vi "PrgEditor.vi"() -> ()   [LabVIEW 2012, in "StimulCtrls.lvlib"]
uses:
  StimulCtrls.lvlib
  SEQPanel.ctl
  Time Slider/Time Slider.xctl
panel:
  in  "Stop Button":bool
  in  "Range Max":dbl=100.0 min=0.0 step=10.0
  in  "Range Min":dbl
  in  "Programs":T1
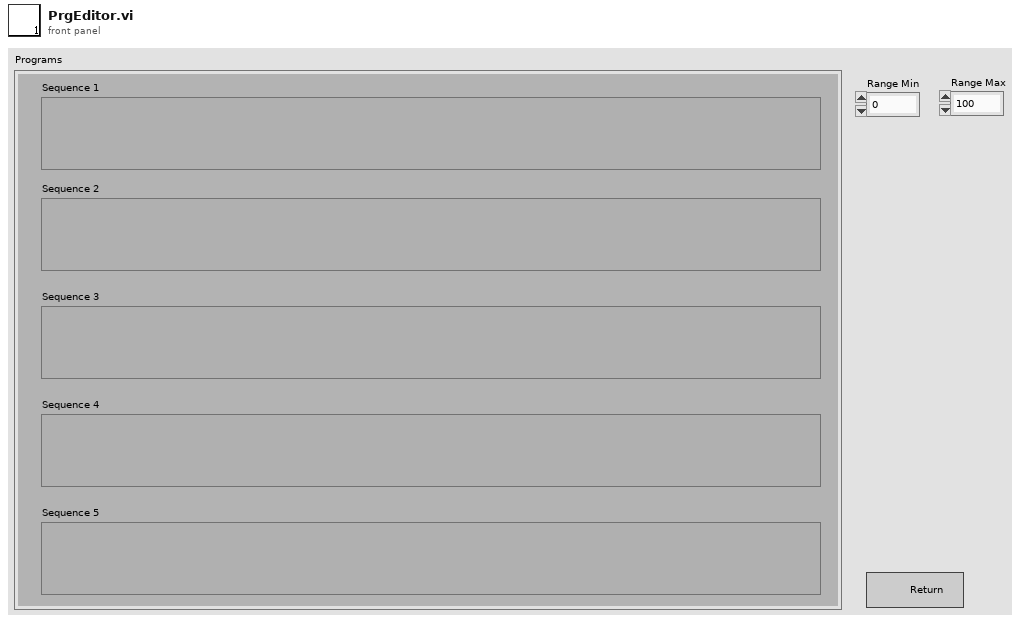
[diagram p1: front panel]
types:
  T1 = typedef "StimulCtrls.lvlib/SEQPanel.ctl" = cluster{"Sequence 1":cluster{"Data":dbl, "Data 2":dbl, "Data 3":dbl}, "Sequence 2":cluster{"Data":dbl, "Data 2":dbl, "Data 3":dbl}, "Sequence 3":cluster{"Data":dbl, "Data 2":dbl, "Data 3":dbl}, "Sequence 4":cluster{"Data":dbl, "Data 2":dbl, "Data 3":dbl}, "Sequence 5":cluster{"Data":dbl, "Data 2":dbl, "Data 3":dbl}}
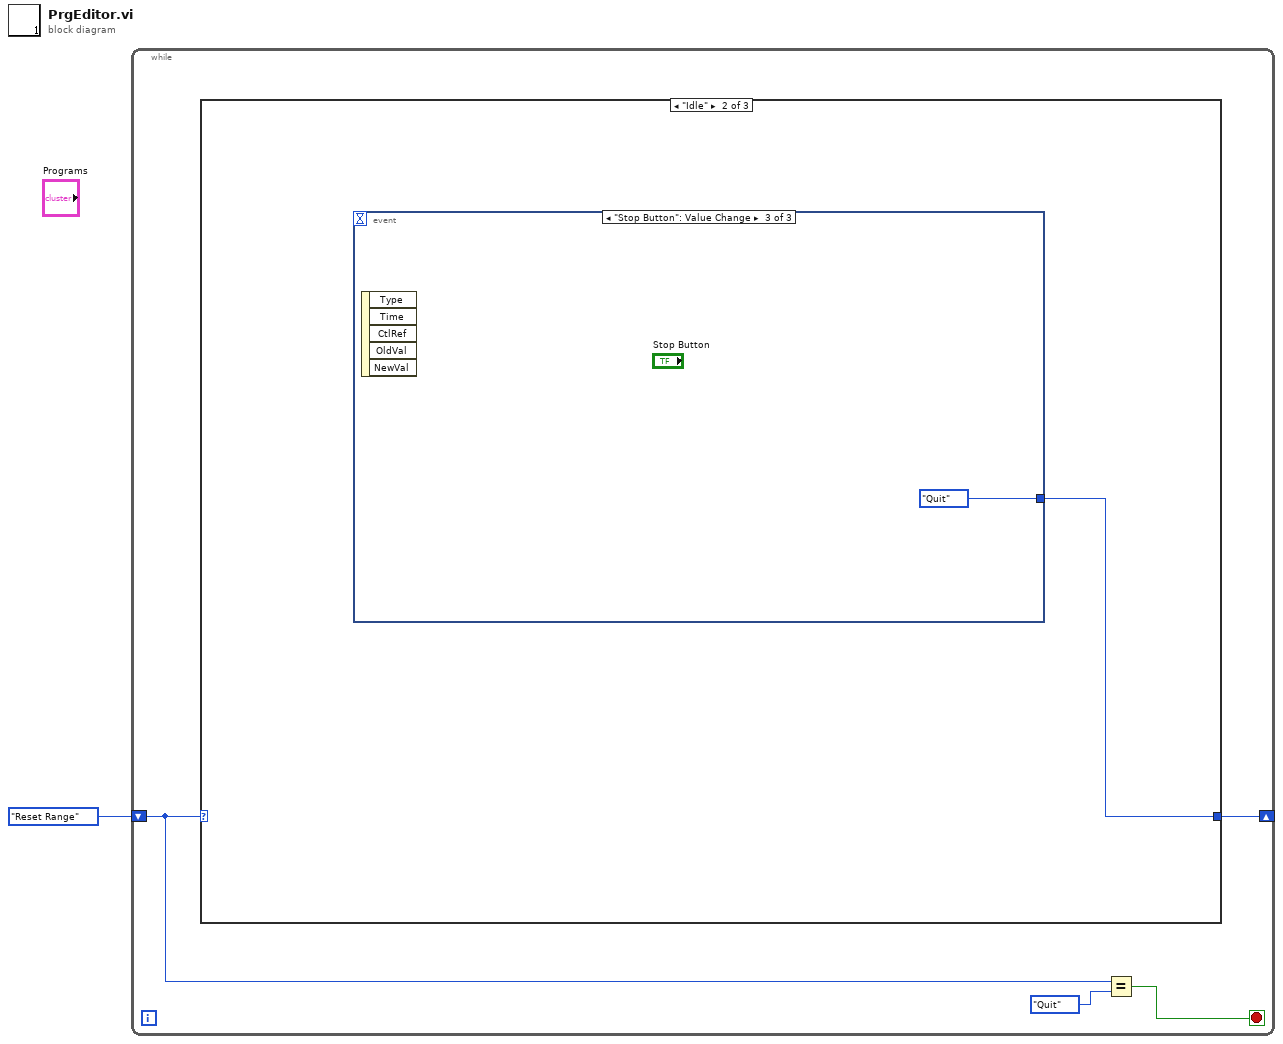
[diagram p0: block diagram]
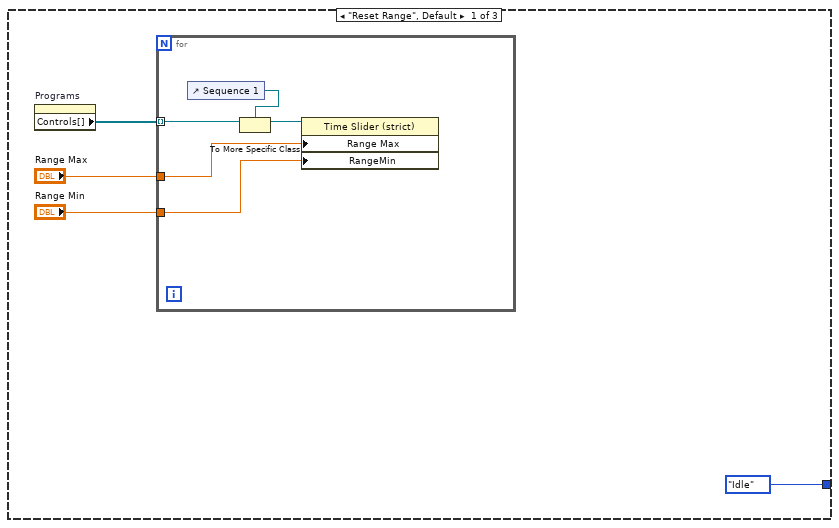
[diagram p2: hidden frame]
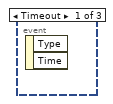
[diagram p3: hidden frame]
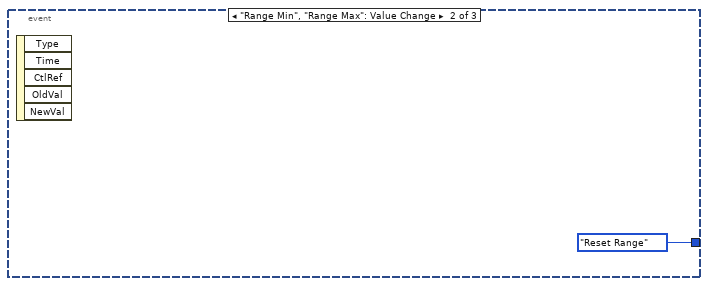
[diagram p4: hidden frame]
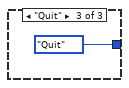
[diagram p5: hidden frame]
diagram:
  n1 = while {
    shift-right: [w5] -> _
    shift-left: enum16{"Reset Range", "Idle", "Quit"}."Reset Range" -> [w3]
    stop <- w2 stop-if-true
    n2 = case shown="\"Idle\"" w3 {
      tunnel: [enum16{"Reset Range", "Idle"}."Idle" w15 enum16{"Reset Range", "Idle", "Quit"}."Quit"] -> w5
      frame "Reset Range", Default {
        n3 = property on="Programs" class="Clust (strict)"() -> ("Controls[]"=w9:refnum<vi>[])  [unwired: 2 in, 2 out]
        n4 = for {
          tunnel: w9 -> [w14] mode=indexing
          tunnel: "Range Min" -> [w10]
          tunnel: "Range Max" -> [w11]
          n5 = control-ref of="Sequence 1"() -> (w13:refnum<vi>)
          n6 = To More Specific Class(target class=w13, reference=w14) -> (specific class reference=w12:refnum<vi>)  [unwired: 1 in, 1 out]
          n7 = property class="Time Slider (strict)"(reference=w12, "Range Max"=w11, "RangeMin"=w10) -> ()  [unwired: 1 in, 2 out]
        }
      }
      frame "Idle" {
        n8 = event shown="[2] \"Stop Button\": Value Change" {
          selector: _ -> [_ _ _]
          dyn-events: _ -> [_ _ _]
          timeout: _ -> [_ _ _]
          tunnel: [_ enum16{"Reset Range", "Idle", "Quit"}."Reset Range" enum16{"Reset Range", "Idle", "Quit"}."Quit"] -> w15
          event Timeout {
            n9 = event-data() -> ()  [unwired: 1 in, 2 out]
          }
          event "Range Min", "Range Max": Value Change {
            n10 = event-data() -> ()  [unwired: 1 in, 5 out]
          }
          event "Stop Button": Value Change {
            n11 = event-data() -> ()  [unwired: 1 in, 5 out]
          }
        }
      }
      frame "Quit" {
      }
    }
    n12 = Equal?(x=w3, y=enum16{"Reset Range", "Idle", "Quit"}."Quit") -> (x = y?=w2:bool)
  }
